vi "Data_Packet_FGV_old.vi"(8 "error in (no error)":errorcluster, 9 "Command":enum16{"Load", "Read", "Write"}(ring), 10 "Packet In":T1, 11 "Packets In":T1[](array[typedef])) -> (0 "error out":errorcluster, 2 "Packet Out":T1, 3 "Packets Out":T1[](array[typedef]))   [LabVIEW 2017]
uses:
  Controls/Packet/Packet.ctl
  Controls/Packet/Packet_Direction.ctl
  Controls/Packet/Packet_Type.ctl
  Controls/Packet/Packet_Priority.ctl
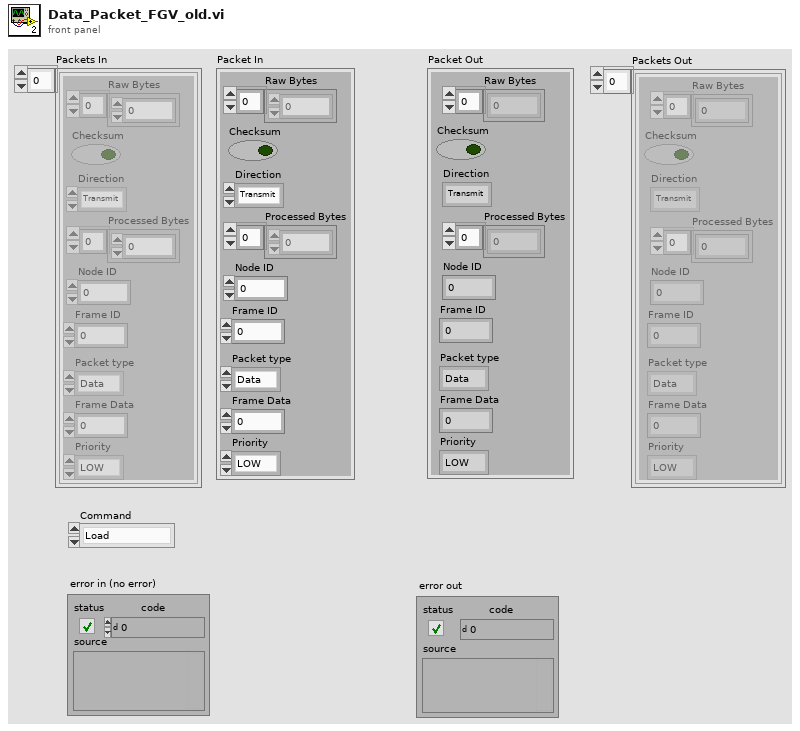
[diagram p1: front panel]
types:
  T1 = typedef "Packet.ctl" = cluster{"Raw Bytes":u8[], "Checksum":bool, "Direction":T2, "Processed Bytes":u8[], "Node ID":u8, "Packet type":T3, "Frame Data":u32, "Priority":T4, "Frame ID":u8}
  T2 = typedef "Packet_Direction.ctl" = enum16{"Transmit", "Receive", "Bidirectional"}
  T3 = typedef "Packet_Type.ctl" = enum16{"Data", "Connection Management", "Remote Request", "Error/Status"}
  T4 = typedef "Packet_Priority.ctl" = enum16{"LOW", "HIGH"}
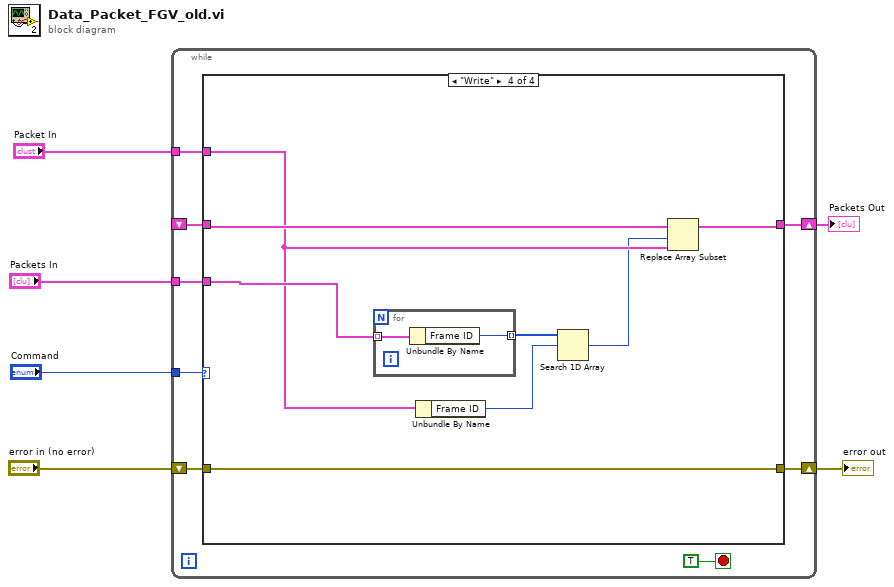
[diagram p0: block diagram]
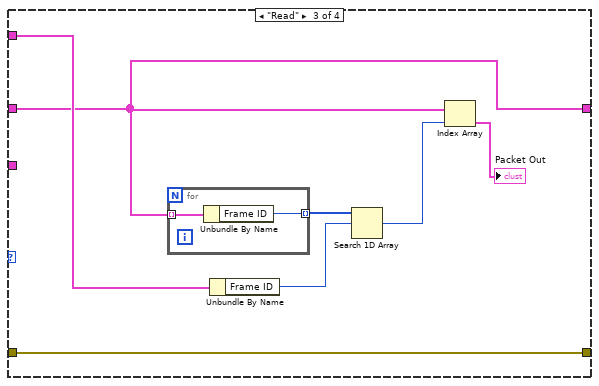
[diagram p4: hidden frame]
diagram:
  n1 = while {
    tunnel: "Packets In" -> [w8]
    tunnel: "Command" -> [w13]
    shift-right: [w11] -> w1
    shift-left: "error in (no error)" -> [w12]
    tunnel: "Packet In" -> [w10]
    shift-right: [w9] -> w2
    shift-left: _ -> [w7]
    stop <- TRUE stop-if-true
    n2 = case shown="\"Write\"" w13 {
      tunnel: w12 -> [w16 w17 w19 w28]
      tunnel: [w16 w17 w19 w28] -> w11
      tunnel: w10 -> [_ _ w24 w31]
      tunnel: [w15 w18 w22 w29] -> w9
      tunnel: w8 -> [_ w18 _ w34]
      tunnel: w7 -> [w15 _ w22 w32]
      frame Default {
      }
      frame "Load" {
      }
      frame "Read" {
        n3 = for {
          tunnel: w22 -> [w27] mode=indexing
          tunnel: [w26] -> w25 mode=indexing
          n4 = Unbundle By Name(w27) -> ("Frame ID"=w26:u8)
        }
        n5 = Unbundle By Name(w24) -> ("Frame ID"=w23:u8)
        n6 = Search 1D Array(1D array=w25, element=w23) -> (index of element=w21:i32)  [unwired: 1 in]
        n7 = Index Array(array=w22, index=w21) -> (element=→"Packet Out":T1)
      }
      frame "Write" {
        n8 = for {
          tunnel: w34 -> [w37] mode=indexing
          tunnel: [w36] -> w35 mode=indexing
          n9 = Unbundle By Name(w37) -> ("Frame ID"=w36:u8)
        }
        n10 = Unbundle By Name(w31) -> ("Frame ID"=w33:u8)
        n11 = Search 1D Array(1D array=w35, element=w33) -> (index of element=w30:i32)  [unwired: 1 in]
        n12 = Replace Array Subset(array=w32, new element=w31, index=w30) -> (w29:T1[])
      }
    }
  }
  "error out" <- w1
  "Packets Out" <- w2
